vi "Pendulum myRIO.vi"() -> ()   [LabVIEW 2018]
uses:
  Model/Target.ctl
  Model/States.ctl
  RL_Ballbalance/LV_Ball_ballance/vi/state.ctl
  <vilib>/Simulation/Scripting/Companion Diagram/SimConfigNode/SimParams.ctl
  <vilib>/Simulation/Scripting/Companion Diagram/SimConfigNode/_simSolvers.ctl
  <vilib>/Simulation/Implementation/Shared/SIMSCR Execution Mode.ctl
  <vilib>/Simulation/Param Hierarchy/Typedefs/SIMPH Param Control Actions.ctl
  <vilib>/Simulation/Implementation/Shared/NILVSim_ParamChanged.vi
  <vilib>/Simulation/Implementation/Shared/NILVSIM_BeginStep.vi
  <vilib>/Simulation/Implementation/Shared/NILVSim_Manager.vi
  <vilib>/Utility/error.llb/Clear Errors.vi
  <vilib>/Simulation/Implementation/Shared/NILVSim_FinalizeModel.vi
  <vilib>/Simulation/Implementation/Shared/SIM Unbundle Sim Info.vi
  <vilib>/Simulation/Implementation/Shared/NILVSim_Initialize.vi
  <vilib>/Simulation/Utility/Implementation/NILVSim Get Time and IsAcceptedStep.vi
  <vilib>/Simulation/Implementation/Shared/SIMSH Read Queue.vi
  <vilib>/Simulation/Implementation/Shared/NILVSim_GetModelError.vi
  <vilib>/Simulation/Implementation/Shared/SIM Bundle Sim Info.vi
  <vilib>/Simulation/Scripting/Companion Diagram/SimConfigNode/SimDog.xnode
  Model/Cart Pendulum Model.vi
  <vilib>/Simulation/Implementation/XNodeFramework/SimXNode/SimX.xnode
  <vilib>/Simulation/Implementation/Shared/NI_SIM_Implementation.lvlib
panel:
  in  "Tab Control":enum32{"config", "run"}(tab)
  in  "move_step":dbl=0.03
  in  "Initial States":T1=[0.0, 0.0, 0.0, 0.0] format="%.4f"
  in  "Target":T2={"Position"=0.0, "Invert"=TRUE} {"Position" min=-0.5 max=0.5 step=0.1 format="%.2g"}
  in  "display tab":enum32{"2D", "3D"}(tab)
  out "Pendulum":picture
  out "3D Picture":refnum<vi>(3d-picture)
  out "status":string
  in  "stop":bool
  out "timer":dbl(knob) scale=0.0..15.0
  in  "start":bool
  out "Seconds":dbl format="%.2f"
  out "In Range?":bool
  out "In Range Sec":dbl format="%.2f"
  out "Done":bool
  out "Off Track":bool
  out "States":T1 format="%.4f"
  out "loop":i32
  in  "left":bool
  in  "right":bool
  in  "pos":dbl(slide) scale=-0.5..0.5
  in  "timeout s":u16=15
  in  "pos_limit":dbl=2.0 format="%#_13g"
  out "read_data":string
  out "connected":bool
  out "dt":u32
  in  "play_type":enum16{"pendulum", "swing up"}(ring)
  out "dt 2":u32
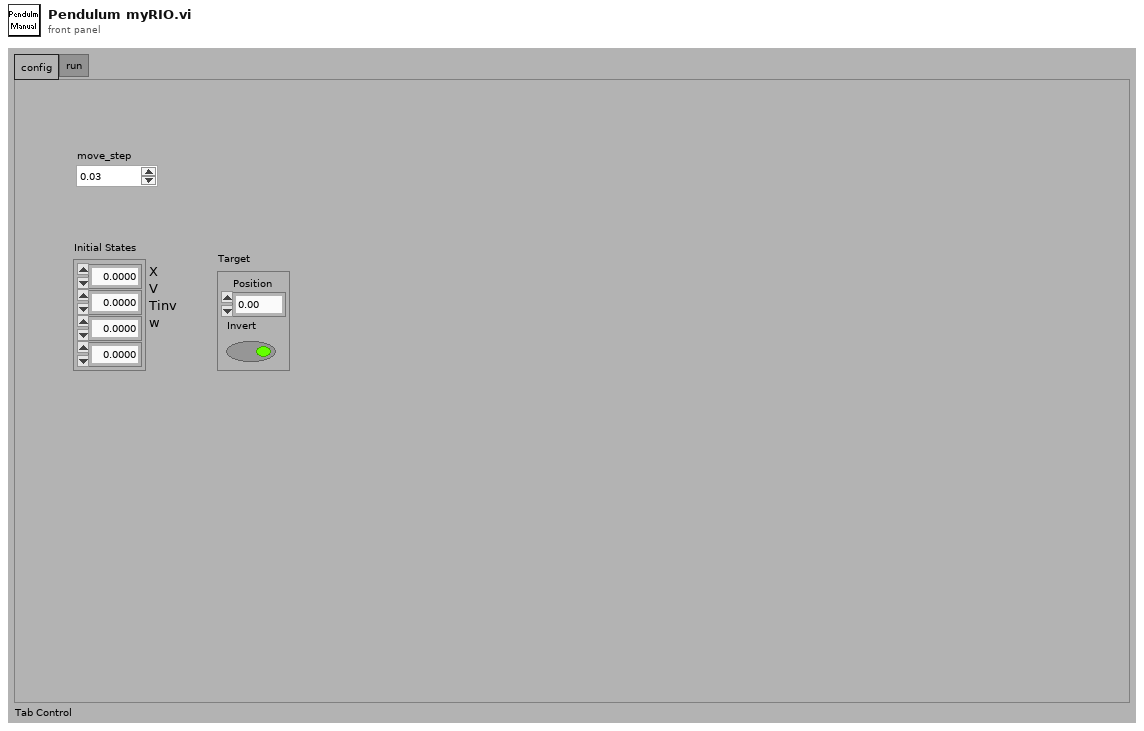
[diagram p1: front panel]
types:
  T1 = typedef "States.ctl" = dbl[]
  T2 = typedef "Target.ctl" = cluster{"Position":dbl, "Invert":bool}
  T3 = typedef "state.ctl" = enum16{"wait for action", "init", "tcp_write", "tct_read", "pause", "wait for python"}
  T4 = typedef "SIMSCR Execution Mode.ctl" = enum16{"Simulate to Completion", "Single Time-Step Simulation (Fixed Step Only)"}
  T5 = typedef "SIMPH Param Control Actions.ctl" = enum16{"get params", "set params"}
  T6 = cluster{"SIMSH Sim Time":dbl, "Integrator 3":cluster{"output":dbl[]}, "Build Array":cluster{"appended array":dbl[]}, "Index Array":cluster{"element":dbl}, "Negate 2":cluster{"-x":dbl}, "Negate":cluster{"-x":dbl}, "Sine & Cosine":cluster{"sin(x)":dbl, "cos(x)":dbl}, "Formula Node":cluster{"dx":dbl, "ddx":dbl, "dT":dbl, "ddT":dbl}}
  T7 = typedef "SimParams.ctl" = cluster{"Initial Time (s)":dbl, "Final Time (s)":dbl, "Step Size (s)":dbl, "ODE Solver":T8, "Minimum Step Size (s)":dbl, "Maximum Step Size (s)":dbl, "Relative Tolerance":dbl, "Absolute Tolerance":dbl, "Software Timing":bool, "Initial Step Size (s)":dbl, "Automatic Fixed Step Size?":bool, "Automatic Discrete Step Size?":bool, "Discrete Step Size (s)":dbl, "Calculate using Time Step":bool, "Solver Wired?":bool, "Prev.Frm.Expected End":u64, "Prev.Frm.Actual End":u64, "Prev.Frm.Finished Late?":bool, "Prev.Iter.Expected End":u64, "Prev.Iter.Actual End":u64, "Prev.Iter.Finished Late?":bool, "Expected Iteration Start":u64, "Actual Iteration Start":u64, "Expected Frame Start":u64, "Actual Frame Start":u64, "Source Name":string, "Name":string, "Period":i64, "Deadline":i64, "Offset":i64, "Start":i64, "Priority":i32, "Timeout":i32, "Processor":i32, "Mode":enum32{"No Change", "Process missed periods, maintain original phase", "Discard missed periods, maintain original phase", "Process missed periods, ignore original phase", "Discard missed periods, ignore original phase"}, "Wakeup reason":enum32{"Normal", "Aborted", "Asynchronous wakeup", "Timing source error", "Timed loop error", "Timeout"}, "Error":errorcluster, "Source Type":string, "Secondary Source Type":string, "Global End Time":u64, "Global Start Time":u64, "Full Solver Reset":bool, "Execution Mode":T4, "Nan/Inf Check":bool, "Custom Solver Library":string, "Solver Is Variable":bool, "custom solver name":string, "Signal Collection Decimation":u32}
  T8 = typedef "_simSolvers.ctl" = enum16{"Runge-Kutta 1 (Euler)", "Runge-Kutta 2", "Runge-Kutta 3", "Runge-Kutta 4", "Runge-Kutta 23 (variable)", "Runge-Kutta 45 (variable)", "BDF (variable)", "Adams-Moulton (variable)", "Rosenbrock (variable)", "Discrete States Only", "SDIRK 4 (variable)", "Radau 5 (variable)", "Radau 9 (variable)", "Radau 13 (variable)", "Radau [Variable Order] (variable)", "Gear's Method (variable)", "Linearizer", "State Query", "Trim Eval", "Custom Solver"}
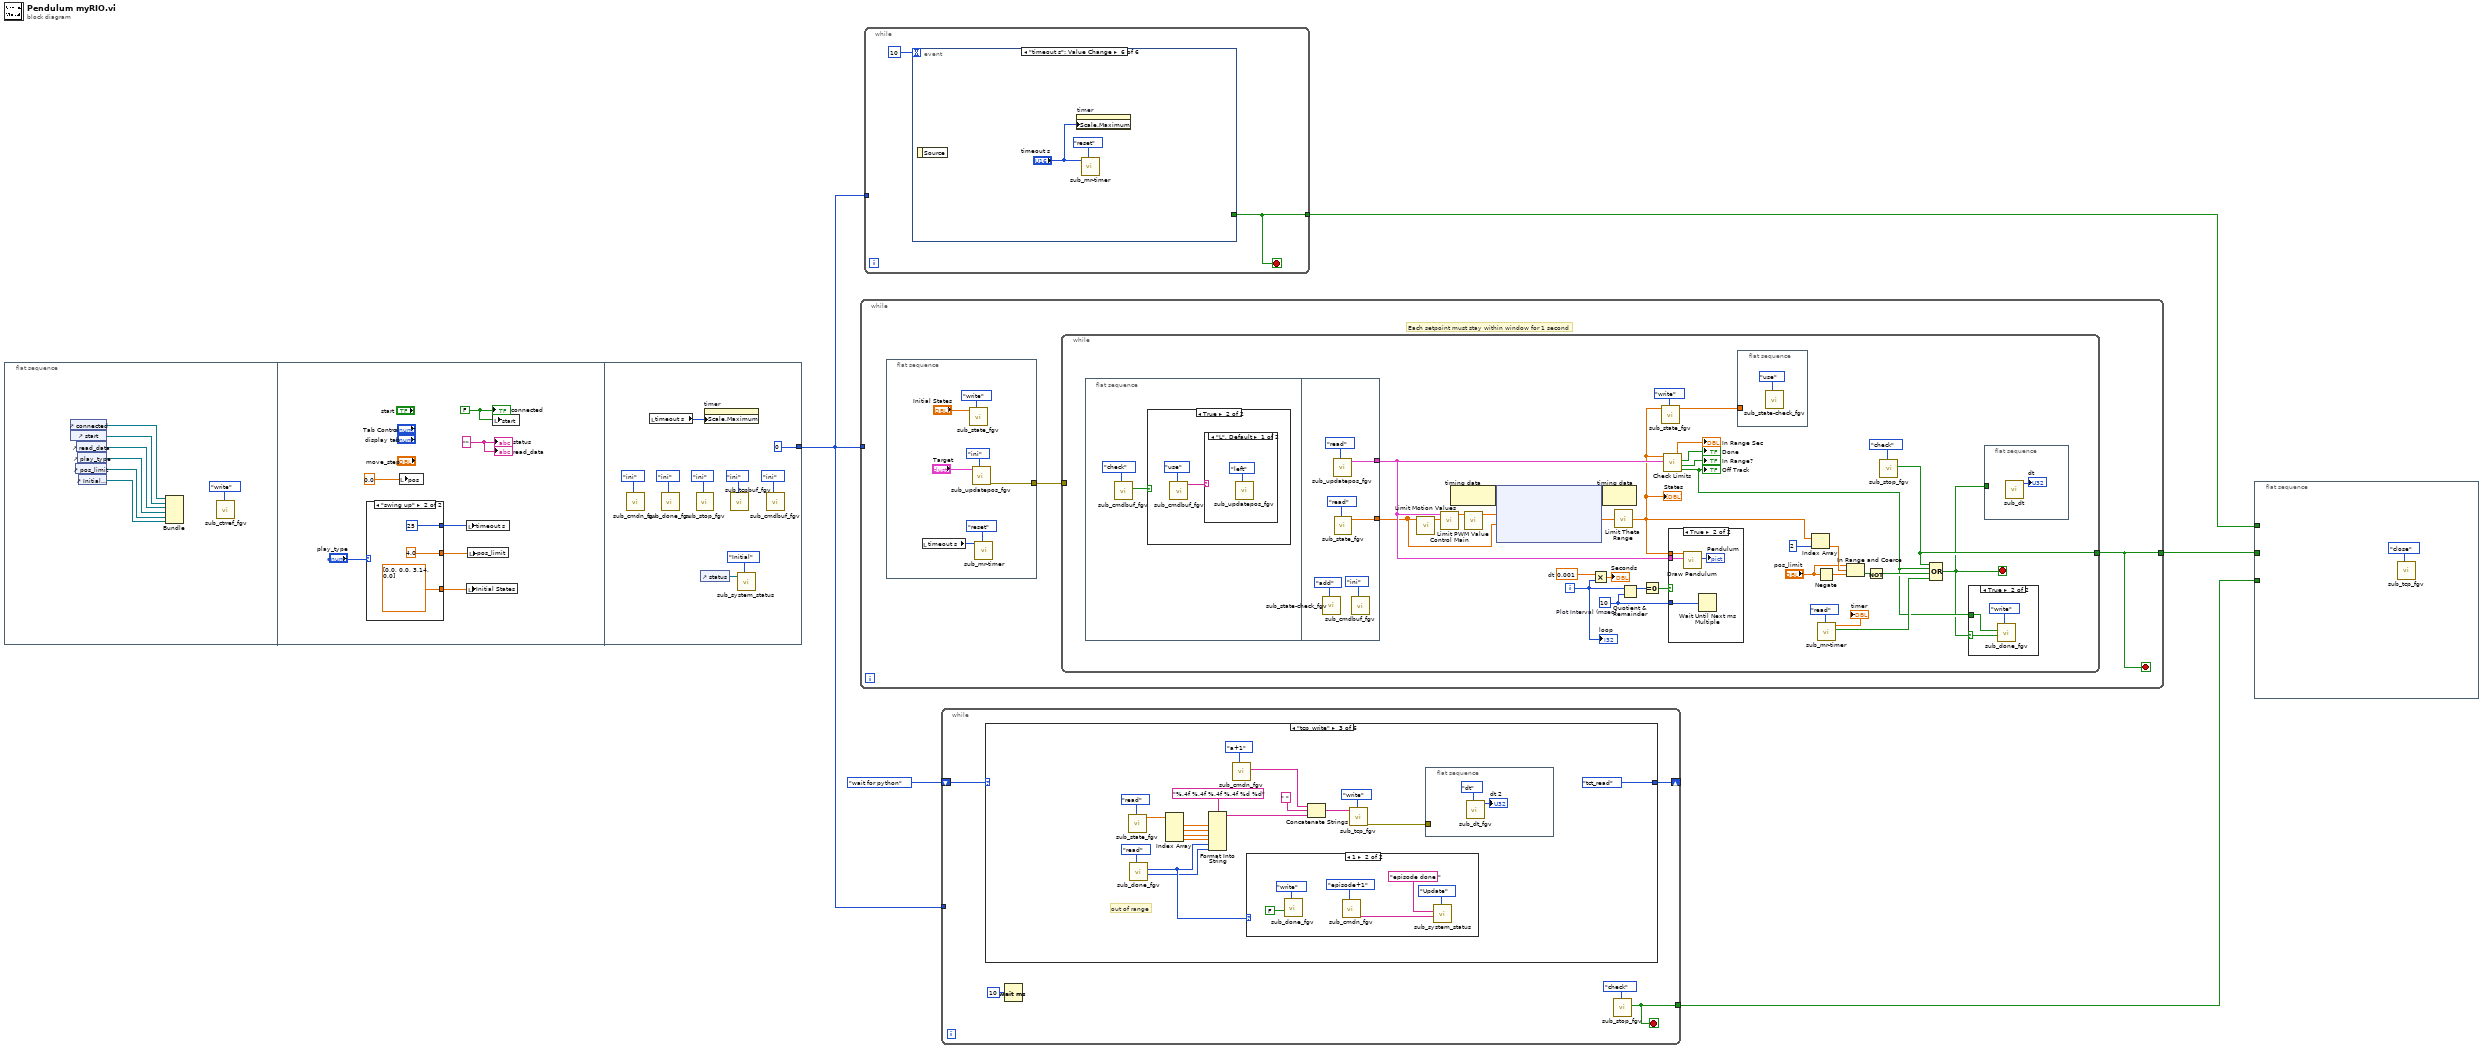
[diagram p0: block diagram]
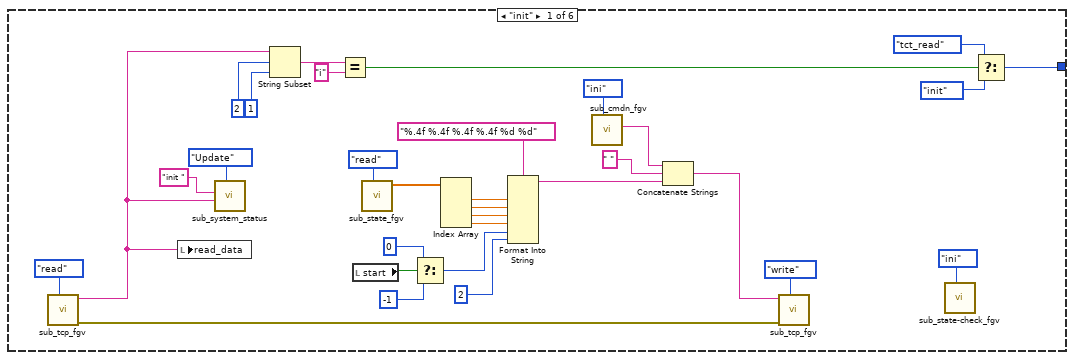
[diagram p2: hidden frame]
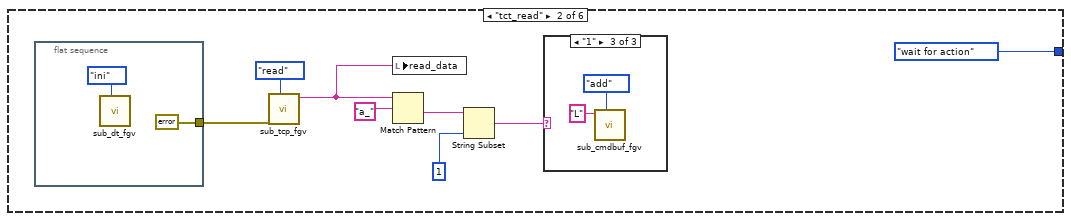
[diagram p3: hidden frame]
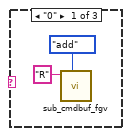
[diagram p4: hidden frame]
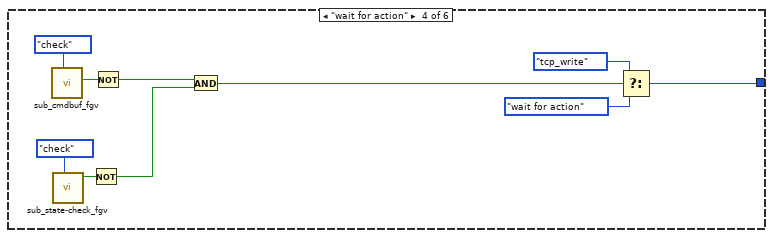
[diagram p7: hidden frame]
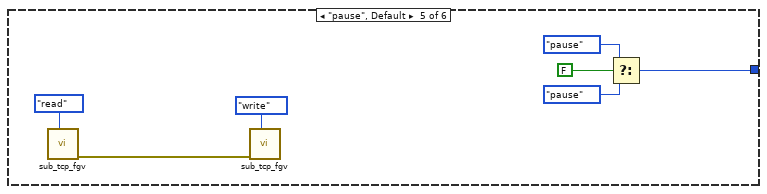
[diagram p8: hidden frame]
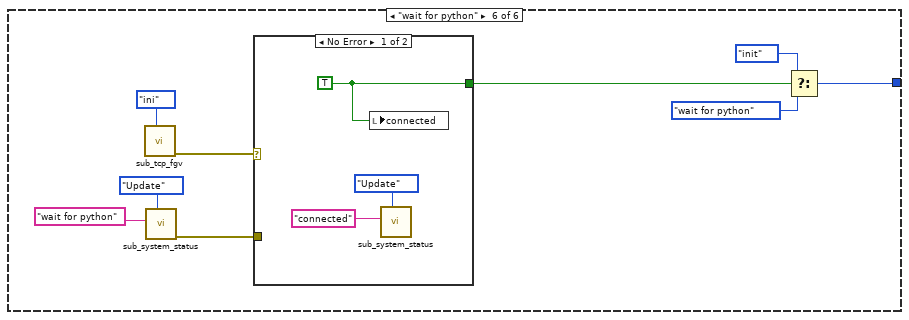
[diagram p9: hidden frame]
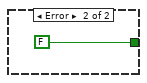
[diagram p10: hidden frame]
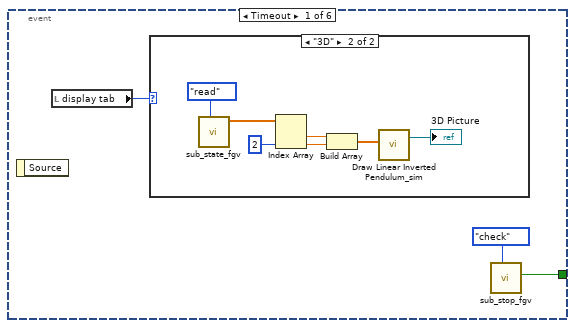
[diagram p11: hidden frame]
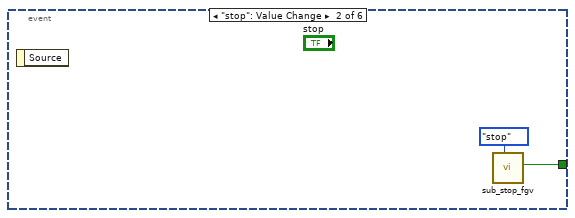
[diagram p13: hidden frame]
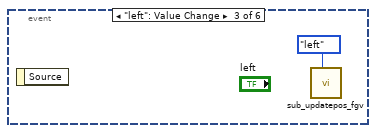
[diagram p14: hidden frame]
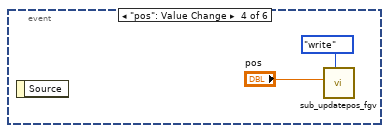
[diagram p15: hidden frame]
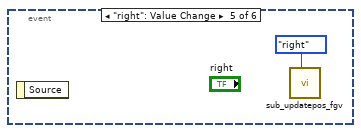
[diagram p16: hidden frame]
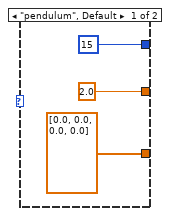
[diagram p17: hidden frame]
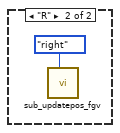
[diagram p20: hidden frame]
diagram:
  n1 = flat-sequence {
    tunnel: [0] -> w1
    frame #0 {
      n2 = control-ref of="connected"() -> (w12:refnum<vi>)
      n3 = control-ref of="start"() -> (w11:refnum<vi>)
      n4 = control-ref of="pos_limit"() -> (w7:refnum<vi>)
      n5 = control-ref of="read_data"() -> (w10:refnum<vi>)
      n6 = control-ref of="play_type"() -> (w8:refnum<vi>)
      n7 = control-ref of="Initial States"() -> (w6:refnum<vi>)
      n8 = Bundle("connected"=w12, "start"=w11, "read_data"=w10, "play_type"=w8, "pos_limit"=w7, "Initial States"=w6) -> ()  [unwired: 1 in, 1 out]
      n9 = call "sub_ctrref_fgv.vi"("cmd"=enum16{"write", "read"}."write") -> ()  [unwired: 10 in, 1 out]
    }
    frame #1 {
      w18 = "" ("status")
      w17 = FALSE ("ini")
      n10 = case shown="\"swing up\"" "play_type" {
        tunnel: [T1 [0.0, 0.0, 0.0, 0.0] ("Initial States") T1 [0.0, 0.0, 3.14, 0.0] ("Initial States")] -> w15
        tunnel: [2.0 ("pos_limit") 4.0 ("pos_limit")] -> w14
        tunnel: [u16 15 ("timeout s") u16 25 ("timeout s")] -> w13
        frame "pendulum", Default {
        }
        frame "swing up" {
        }
      }
      n11 = local write "pos"(0.0 ("pos")) -> ()
      n12 = local write "timeout s"(w13) -> ()
      n13 = local write "Initial States"(w15) -> ()
      n14 = local write "pos_limit"(w14) -> ()
      n15 = local write "start"(w17) -> ()
      "status" <- w18
      "connected" <- w17
      "read_data" <- w18
    }
    frame #2 {
      n16 = call "sub_cmdn_fgv.vi"("cmd"=enum16{"ini", "a+1", "episode+1", "read"}."ini") -> ()  [unwired: 7 in, 4 out]
      n17 = local read "timeout s"() -> (w26:u16)
      n18 = call "sub_done_fgv.vi"("cmd"=enum16{"ini", "write", "read"}."ini") -> ()  [unwired: 9 in, 2 out]
      n19 = call "sub_stop_fgv.vi"("cmd"=enum16{"ini", "check", "stop"}."ini") -> ()  [unwired: 10 in, 1 out]
      n20 = control-ref of="status"() -> (w31:refnum<vi>)
      n21 = property on="timer" class="Knob (strict)"("Scale.Maximum"=w26) -> ()  [unwired: 2 in, 2 out]
      n22 = call "sub_tcpbuf_fgv.vi"("cmd"=enum16{"ini", "add", "use", "check"}."ini") -> ()  [unwired: 8 in, 3 out]
      n23 = call "sub_system_status.vi"("Mode"=enum16{"Initial", "Update", "Clear"}."Initial", "System Log"=w31) -> ()  [unwired: 9 in, 1 out]
      n24 = call "sub_cmdbuf_fgv.vi"("cmd"=enum16{"ini", "add", "use", "check"}."ini") -> ()  [unwired: 9 in, 2 out]
    }
  }
  n25 = while {
    tunnel: w1 -> [_]
    tunnel: [w36] -> w3
    stop <- w36 stop-if-true
    # "Each setpoint must stay within window for 1 second"
    n26 = flat-sequence {
      tunnel: [w37] -> w35
      frame #0 {
        n27 = local read "timeout s"() -> (w38:u16)
        n28 = call "sub_state_fgv.vi"("cmd"=enum16{"read", "write"}."write", "Initial States"="Initial States") -> ()  [unwired: 9 in, 1 out]
        n29 = call "sub_updatepos_fgv.vi"("cmd"=enum16{"left", "right", "ini", "read", "write"}."ini", "Target"="Target") -> ("error out"=w37:errorcluster)  [unwired: 8 in, 1 out]
        n30 = call "sub_mr-timer.vi"("cmd"=enum16{"reset", "read"}."reset", "limit s"=w38) -> ()  [unwired: 8 in, 2 out]
      }
    }
    n31 = while {
      tunnel: [w48] -> w36
      tunnel: w35 -> [_]
      i -> [w73]
      stop <- w44 stop-if-true
      w68 = 0.001  # dt
      w69 = u32 10  # Plot Interval (msec)
      n32 = flat-sequence {
        tunnel: [w92] -> w56
        tunnel: [w90] -> w52
        frame #0 {
          n33 = call "sub_cmdbuf_fgv.vi"("cmd"=enum16{"ini", "add", "use", "check"}."check") -> ("data"=w82:bool)  [unwired: 9 in, 1 out]
          n34 = case shown="True" w82 {
            frame False {
            }
            frame True {
              n35 = call "sub_cmdbuf_fgv.vi"("cmd"=enum16{"ini", "add", "use", "check"}."use") -> ("element"=w84:string)  [unwired: 9 in, 1 out]
              n36 = case shown="\"L\", Default" w84 {
                frame "L", Default {
                  n37 = call "sub_updatepos_fgv.vi"("cmd"=enum16{"left", "right", "ini", "read", "write"}."left") -> ()  [unwired: 9 in, 2 out]
                }
                frame "R" {
                  n38 = call "sub_updatepos_fgv.vi"("cmd"=enum16{"left", "right", "ini", "read", "write"}."right") -> ()  [unwired: 9 in, 2 out]
                }
              }
            }
          }
        }
        frame #1 {
          n39 = call "sub_state-check_fgv.vi"("cmd"=enum16{"ini", "add", "use", "check"}."add") -> ()  [unwired: 9 in, 2 out]
          n40 = call "sub_updatepos_fgv.vi"("cmd"=enum16{"left", "right", "ini", "read", "write"}."read") -> ("Target_out"=w92:T2)  [unwired: 9 in, 1 out]
          n41 = call "sub_state_fgv.vi"("cmd"=enum16{"read", "write"}."read") -> ("state_out"=w90:dbl[])  [unwired: 10 in]
          n42 = call "sub_cmdbuf_fgv.vi"("cmd"=enum16{"ini", "add", "use", "check"}."ini") -> ()  [unwired: 9 in, 2 out]
        }
      }
      n43 = call "Limit Motion Values.vi"("States In"=w52) -> ("States Out"=w67:T1)  [unwired: 10 in]
      n44 = call "Control Main.vi"("States"=w67, "Target"=w56) -> ("PWM"=w64:dbl)  [unwired: 9 in]
      n45 = node-c288() -> (w66:variant)  [unwired: 1 in]
      n46 = call "Limit PWM Value.vi"("PWM In"=w64) -> ("PWM Out"=w63:dbl)  [unwired: 10 in]
      n47 = node-c254 ("Control & Simulation Loop 2")(w66, w63, w52) -> (w65:variant, w62:dbl[])
      n48 = Multiply(x=w68, y=w73) -> (x*y=→"Seconds":dbl)
      n49 = node-c288(w65) -> ()  [unwired: 1 out]
      n50 = call "Limit Theta Range.vi"("States In"=w62) -> ("States Out"=w54:T1)
      "States" <- w54
      n51 = Quotient & Remainder(x=w73, y=w69) -> (x-y*floor(x/y)=w76:u32)  [unwired: 1 out]
      n52 = Equal To 0?(x=w76) -> (x = 0?=w75:bool)
      n53 = call "sub_state_fgv.vi"("cmd"=enum16{"read", "write"}."write", "Initial States"=w54) -> ("state_out"=w46:dbl[])  [unwired: 9 in]
      n54 = call "Check Limits.vi"("Target"=w56, "States"=w54) -> ("Off Track"=w45:bool, "In Range"=→"In Range?":bool, "Done"=→"Done":bool, "In Range Seconds"=→"In Range Sec":dbl)  [unwired: 3 in]
      "Off Track" <- w45
      n55 = case shown="True" w75 {
        tunnel: w54 -> [_ w329]
        tunnel: w56 -> [_ w328]
        tunnel: w69 -> [_ w327]
        frame False {
        }
        frame True {
          n56 = call "Draw Pendulum.vi"("Target"=w328, "States In"=w329) -> ("Picture"=→"Pendulum":picture)  [unwired: 1 in, 8 out]
          n57 = Wait Until Next ms Multiple(millisecond multiple=w327) -> ()  [unwired: 1 out]
        }
      }
      n58 = flat-sequence {
        tunnel: w46 -> [_]
        frame #0 {
          n59 = call "sub_state-check_fgv.vi"("cmd"=enum16{"ini", "add", "use", "check"}."use") -> ()  [unwired: 9 in, 2 out]
        }
      }
      n60 = Index Array(array=w54, index=2) -> (element=w59:dbl)
      n61 = Negate(x="pos_limit") -> (-x=w50:dbl)
      n62 = call "sub_mr-timer.vi"("cmd"=enum16{"reset", "read"}."read") -> ("timeout"=w55:bool, "time"=→"timer":dbl)  [unwired: 9 in]
      n63 = In Range and Coerce(upper limit="pos_limit", x=w59, lower limit=w50) -> (In Range?=w49:bool)  [unwired: 1 out]
      n64 = Not(x=w49) -> (.not. x?=w47:bool)
      n65 = call "sub_stop_fgv.vi"("cmd"=enum16{"ini", "check", "stop"}."check") -> ("status"=w48:bool)  [unwired: 10 in]
      n66 = Compound Arithmetic op=OR(w48, w45, w47, w55) -> (w44:bool)
      n67 = case shown="True" w44 {
        selector: w44 -> [_ w81]
        tunnel: w45 -> [_ w79]
        frame False {
        }
        frame True {
          n68 = call "sub_done_fgv.vi"("cmd"=enum16{"ini", "write", "read"}."write", "input"=w81, "off_track"=w79) -> ()  [unwired: 7 in, 2 out]
        }
      }
      n69 = flat-sequence {
        tunnel: w44 -> [_]
        frame #0 {
          n70 = call "sub_dt.vi"() -> ("dt"=→"dt":u32)  [unwired: 11 in]
        }
      }
      "loop" <- w73
    }
  }
  n71 = while {
    tunnel: w1 -> [_]
    tunnel: [w332] -> w4
    stop <- w332 stop-if-true
    n72 = event shown="[5] \"timeout s\": Value Change" {
      selector: _ -> [_ _ _ _ _ _]
      dyn-events: _ -> [_ _ _ _ _ _]
      timeout: 10 -> [_ _ _ _ _ _]
      tunnel: [w334 w343 _ _ _ _] -> w332
      event Timeout {
        n73 = event-data() -> ()  [unwired: 1 in, 1 out]
        n74 = local read "display tab"() -> (w333:enum32{"2D", "3D"})
        n75 = case shown="\"3D\"" w333 {
          frame "2D", Default {
          }
          frame "3D" {
            n76 = call "sub_state_fgv.vi"("cmd"=enum16{"read", "write"}."read") -> ("state_out"=w338:dbl[])  [unwired: 10 in]
            n77 = Index Array(array=w338, index #2=2 ("index")) -> (element #1=w339:dbl, element #2=w340:dbl)  [unwired: 1 in]
            n78 = Build Array(w339, w340) -> (w341:dbl[])
            n79 = call "Draw Linear Inverted Pendulum_sim.vi"("Linear Pos and Angle"=w341) -> ("Scene.New Object"=→"3D Picture":refnum<vi>)  [unwired: 4 in, 1 out]
          }
        }
        n80 = call "sub_stop_fgv.vi"("cmd"=enum16{"ini", "check", "stop"}."check") -> ("status"=w334:bool)  [unwired: 10 in]
      }
      event "stop": Value Change {
        n81 = event-data() -> ()  [unwired: 1 in, 1 out]
        n82 = call "sub_stop_fgv.vi"("cmd"=enum16{"ini", "check", "stop"}."stop") -> ("status"=w343:bool)  [unwired: 10 in]
      }
      event "left": Value Change {
        n83 = event-data() -> ()  [unwired: 1 in, 1 out]
        n84 = call "sub_updatepos_fgv.vi"("cmd"=enum16{"left", "right", "ini", "read", "write"}."left") -> ()  [unwired: 9 in, 2 out]
      }
      event "pos": Value Change {
        n85 = event-data() -> ()  [unwired: 1 in, 1 out]
        n86 = call "sub_updatepos_fgv.vi"("cmd"=enum16{"left", "right", "ini", "read", "write"}."write", "pos"="pos") -> ()  [unwired: 8 in, 2 out]
      }
      event "right": Value Change {
        n87 = event-data() -> ()  [unwired: 1 in, 1 out]
        n88 = call "sub_updatepos_fgv.vi"("cmd"=enum16{"left", "right", "ini", "read", "write"}."right") -> ()  [unwired: 9 in, 2 out]
      }
      event "timeout s": Value Change {
        n89 = event-data() -> ()  [unwired: 1 in, 1 out]
        n90 = property on="timer" class="Knob (strict)"("Scale.Maximum"="timeout s") -> ()  [unwired: 2 in, 2 out]
        n91 = call "sub_mr-timer.vi"("cmd"=enum16{"reset", "read"}."reset", "limit s"="timeout s") -> ()  [unwired: 8 in, 2 out]
      }
    }
  }
  n92 = while {
    tunnel: w1 -> [_]
    shift-right: [w351] -> _
    shift-left: state."wait for python" ("state") -> [w352]
    tunnel: [w353] -> w2
    stop <- w353 stop-if-true
    n93 = case shown="\"tcp_write\"" w352 {
      tunnel: [w387 state."wait for action" ("state") state."tct_read" ("state") w435 w442 w449] -> w351
      frame "init" {
        n94 = call "sub_tcp_fgv.vi"("cmd"=enum16{"ini", "read", "write", "close"}."read") -> ("error out"=w357:errorcluster, "read_data"=w358:string)  [unwired: 8 in, 1 out]
        n95 = local write "read_data"(w358) -> ()
        n96 = call "sub_system_status.vi"("Mode"=enum16{"Initial", "Update", "Clear"}."Update", "content"=w358, "title"="init " ("String in")) -> ()  [unwired: 8 in, 1 out]
        n97 = String Subset(string=w358, offset (0)=2, length (rest)=1 ("length (rest)")) -> (substring=w380:string)
        n98 = Equal?(x=w380, y="i") -> (x = y?=w360:bool)
        n99 = local read "start"() -> (w359:bool)
        n100 = call "sub_state_fgv.vi"("cmd"=enum16{"read", "write"}."read") -> ("state_out"=w378:dbl[])  [unwired: 10 in]
        n101 = Select(t=i8 0, s=w359, f=i8 -1) -> (s? t:f=w372:i8)
        n102 = Index Array(array=w378) -> (element #1=w377:dbl, element #2=w376:dbl, element #3=w375:dbl, element #4=w374:dbl)  [unwired: 4 in]
        n103 = Format Into String(format string="%.4f %.4f %.4f %.4f %d %d" ("포맷 문자열"), w377, w376, w375, w374, w372, i8 2 ("입력 6")) -> (resulting string=w373:string)  [unwired: 2 in, 1 out]
        n104 = call "sub_cmdn_fgv.vi"("cmd"=enum16{"ini", "a+1", "episode+1", "read"}."ini") -> ("action_str"=w363:string)  [unwired: 7 in, 3 out]
        n105 = Concatenate Strings(w363, " " ("구분 문자 (탭)"), w373) -> (w367:string)
        n106 = call "sub_tcp_fgv.vi"("cmd"=enum16{"ini", "read", "write", "close"}."write", "error in (no error)"=w357, "write_data"=w367) -> ()  [unwired: 6 in, 3 out]
        n107 = call "sub_state-check_fgv.vi"("cmd"=enum16{"ini", "add", "use", "check"}."ini") -> ()  [unwired: 9 in, 2 out]
        n108 = Select(t=state."tct_read" ("state"), s=w360, f=state."init" ("state")) -> (s? t:f=w387:T3)
      }
      frame "tct_read" {
        n109 = flat-sequence {
          tunnel: [errorcluster {"status"=FALSE, "code"=0, "source"=""} ("error out")] -> w388
          frame #0 {
            n110 = call "sub_dt_fgv.vi"("cmd"=enum16{"ini", "dt"}."ini") -> ()  [unwired: 10 in, 1 out]
          }
        }
        n111 = call "sub_tcp_fgv.vi"("cmd"=enum16{"ini", "read", "write", "close"}."read", "error in (no error)"=w388) -> ("read_data"=w394:string)  [unwired: 7 in, 2 out]
        n112 = local write "read_data"(w394) -> ()
        n113 = Match Pattern(string=w394, regular expression="a_") -> (after substring=w392:string)  [unwired: 1 in, 3 out]
        n114 = String Subset(string=w392, length (rest)=1 ("length (rest)")) -> (substring=w390:string)  [unwired: 1 in]
        n115 = case shown="\"1\"" w390 {
          frame "0" {
            n116 = call "sub_cmdbuf_fgv.vi"(7:"cmd"=enum16{"ini", "add", "use", "check"}."add" ("cmd"), 11:"cmd"="R" ("cmd")) -> ()  [unwired: 8 in, 2 out]
          }
          frame "-1", Default {
          }
          frame "1" {
            n117 = call "sub_cmdbuf_fgv.vi"(7:"cmd"=enum16{"ini", "add", "use", "check"}."add" ("cmd"), 11:"cmd"="L" ("cmd")) -> ()  [unwired: 8 in, 2 out]
          }
        }
      }
      frame "tcp_write" {
        # "out of range"
        n118 = call "sub_state_fgv.vi"("cmd"=enum16{"read", "write"}."read") -> ("state_out"=w417:dbl[])  [unwired: 10 in]
        n119 = call "sub_done_fgv.vi"("cmd"=enum16{"ini", "write", "read"}."read") -> ("range_val"=w403:i32, "done_val"=w404:i32)  [unwired: 9 in]
        n120 = Index Array(array=w417) -> (element #1=w416:dbl, element #2=w415:dbl, element #3=w414:dbl, element #4=w413:dbl)  [unwired: 4 in]
        n121 = Format Into String(format string="%.4f %.4f %.4f %.4f %d %d" ("포맷 문자열"), w416, w415, w414, w413, w404, w403) -> (resulting string=w412:string)  [unwired: 2 in, 1 out]
        n122 = call "sub_cmdn_fgv.vi"("cmd"=enum16{"ini", "a+1", "episode+1", "read"}."a+1") -> ("action_str"=w407:string)  [unwired: 7 in, 3 out]
        n123 = case shown="1" w404 {
          frame 0, Default {
          }
          frame 1 {
            n124 = call "sub_done_fgv.vi"("cmd"=enum16{"ini", "write", "read"}."write", "input"=FALSE) -> ()  [unwired: 8 in, 2 out]
            n125 = call "sub_cmdn_fgv.vi"("cmd"=enum16{"ini", "a+1", "episode+1", "read"}."episode+1") -> ("episode_str"=w423:string)  [unwired: 7 in, 3 out]
            n126 = call "sub_system_status.vi"("Mode"=enum16{"Initial", "Update", "Clear"}."Update", "content"=w423, "title"="episode done ") -> ()  [unwired: 8 in, 1 out]
          }
        }
        n127 = Concatenate Strings(w407, " " ("구분 문자 (탭)"), w412) -> (w419:string)
        n128 = call "sub_tcp_fgv.vi"("cmd"=enum16{"ini", "read", "write", "close"}."write", "write_data"=w419) -> ("error out"=w402:errorcluster)  [unwired: 7 in, 2 out]
        n129 = flat-sequence {
          tunnel: w402 -> [_]
          frame #0 {
            n130 = call "sub_dt_fgv.vi"("cmd"=enum16{"ini", "dt"}."dt") -> ("dt"=→"dt 2":u32)  [unwired: 10 in]
          }
        }
      }
      frame "wait for action" {
        n131 = call "sub_cmdbuf_fgv.vi"("cmd"=enum16{"ini", "add", "use", "check"}."check") -> ("data"=w431:bool)  [unwired: 9 in, 1 out]
        n132 = call "sub_state-check_fgv.vi"("cmd"=enum16{"ini", "add", "use", "check"}."check") -> ("data"=w432:bool)  [unwired: 9 in, 1 out]
        n133 = Not(x=w432) -> (.not. x?=w428:bool)
        n134 = Not(x=w431) -> (.not. x?=w429:bool)
        n135 = And(x=w429, y=w428) -> (x .and. y?=w430:bool)
        n136 = Select(t=state."tcp_write" ("state"), s=w430, f=state."wait for action") -> (s? t:f=w435:T3)
      }
      frame "pause", Default {
        n137 = call "sub_tcp_fgv.vi"("cmd"=enum16{"ini", "read", "write", "close"}."read") -> ("error out"=w439:errorcluster)  [unwired: 8 in, 2 out]
        n138 = call "sub_tcp_fgv.vi"("cmd"=enum16{"ini", "read", "write", "close"}."write", "error in (no error)"=w439) -> ()  [unwired: 7 in, 3 out]
        n139 = Select(t=state."pause" ("f"), s=FALSE, f=state."pause") -> (s? t:f=w442:T3)
      }
      frame "wait for python" {
        n140 = call "sub_tcp_fgv.vi"("cmd"=enum16{"ini", "read", "write", "close"}."ini") -> ("error out"=w450:errorcluster)  [unwired: 8 in, 2 out]
        n141 = call "sub_system_status.vi"("Mode"=enum16{"Initial", "Update", "Clear"}."Update", "title"="wait for python" ("String in")) -> ("error out"=w445:errorcluster)  [unwired: 9 in]
        n142 = case shown="No Error" w450 {
          tunnel: [w454 FALSE ("s")] -> w448
          tunnel: w445 -> [_ _]
          frame No Error {
            w454 = TRUE ("s")
            n143 = local write "connected"(w454) -> ()
            n144 = call "sub_system_status.vi"("Mode"=enum16{"Initial", "Update", "Clear"}."Update", "title"="connected" ("String in")) -> ()  [unwired: 9 in, 1 out]
          }
          frame Error {
          }
        }
        n145 = Select(t=state."init" ("f"), s=w448, f=state."wait for python") -> (s? t:f=w449:T3)
      }
    }
    n146 = Wait (ms)(milliseconds to wait=u32 10) -> ()  [unwired: 1 out]
    n147 = call "sub_stop_fgv.vi"("cmd"=enum16{"ini", "check", "stop"}."check") -> ("status"=w353:bool)  [unwired: 10 in]
  }
  n148 = flat-sequence {
    tunnel: w4 -> [_]
    tunnel: w3 -> [_]
    tunnel: w2 -> [_]
    frame #0 {
      n149 = call "sub_tcp_fgv.vi"("cmd"=enum16{"ini", "read", "write", "close"}."close") -> ()  [unwired: 8 in, 3 out]
    }
  }
